vi "Arduino_Timed_Release.vi"(2 "Time to hold source ON (microseconds)":u32=1000000 format="%.0g", 3 "Time to hold source OFF (microseconds)":u32=1000000 format="%.0g", 4 "Number of cycles":u16=1) -> (0 "error out":errorcluster, 1 "Completed cycles":u16=5)   [LabVIEW 2014]
uses:
  ADAM Client/Sub VIs/ADAM Controls/Update_scan_value.ctl
  Globals/Gas_management_global.vi
  Arduino_common/Arduino_comms_Global.vi
panel:
  in  "Device index":i32
  out "bytes sent":u32=12
  out "write buffer":string
  # "(enter 0 for continuous ON)*"
  # "(enter 0 for continuous OFF)*"
  # "Paul Nathan, 18/06/2013, 02/05/2014, 12/08/2014, 03/10/2014, 10/12/2014"
  # "*until next communication. Ensure n cycles is 1 for these special operations."
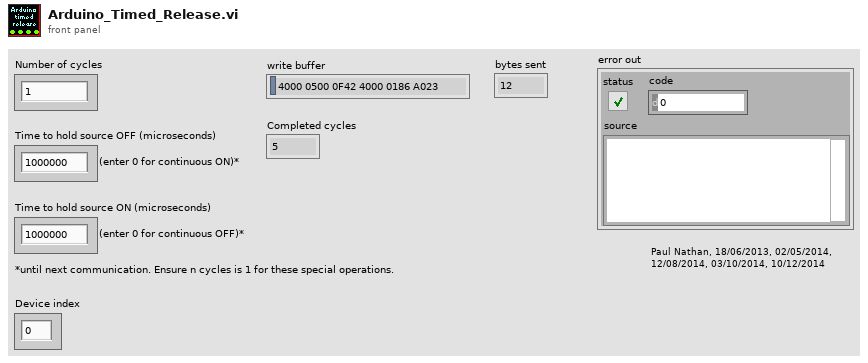
[diagram p1: front panel]
types:
  T1 = typedef "Update_scan_value.ctl" = cluster{"Channel Name":string, "New Value":dbl}
  T2 = typedef "Arduino Config & resource typedef.ctl" = cluster{"VISA resource name":refnum<visa-resource-name>, "baud rate (bps)":u32, "timeout (ms)":u32, "data bits":u16, "parity":enum16{"None", "Odd", "Even", "Mark", "Space"}, "stop bits (10: 1 bit)":u16, "flow control":u16, "termination char (hex)":u8, "Enable Termination Char":bool, "byte count":u32, "Resource locked?":bool}
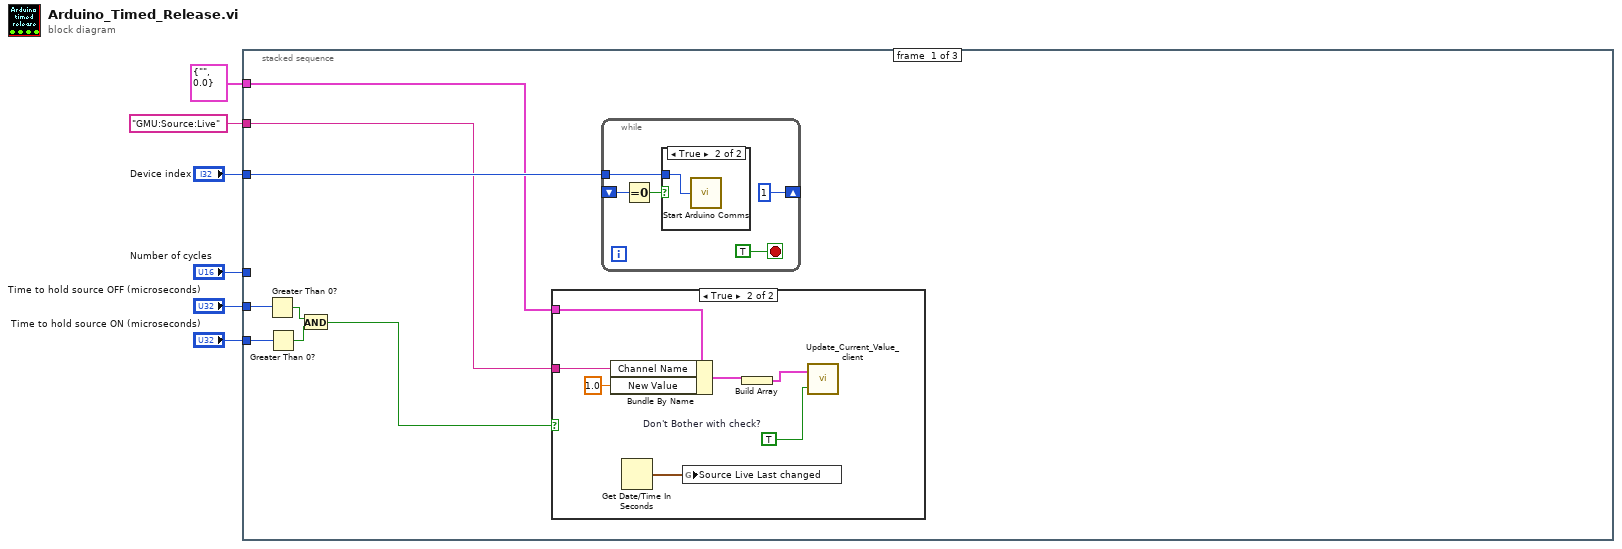
[diagram p0: block diagram]
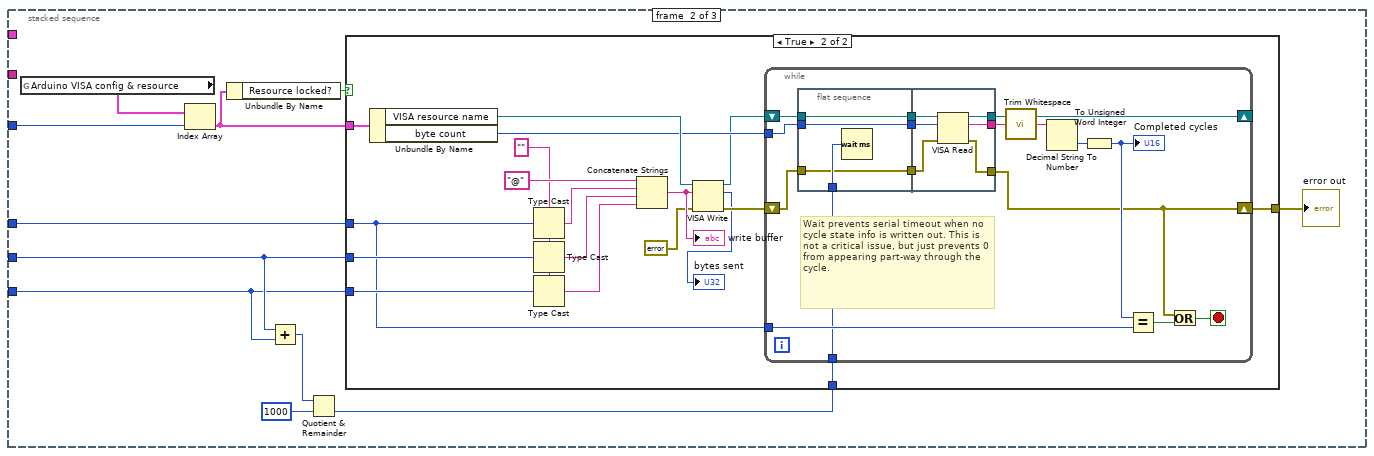
[diagram p4: hidden frame]
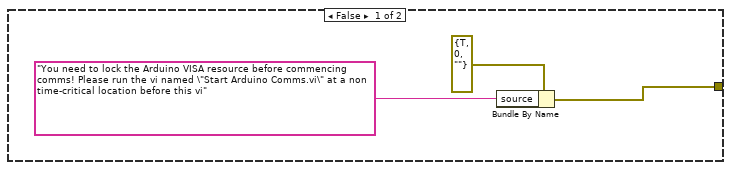
[diagram p5: hidden frame]
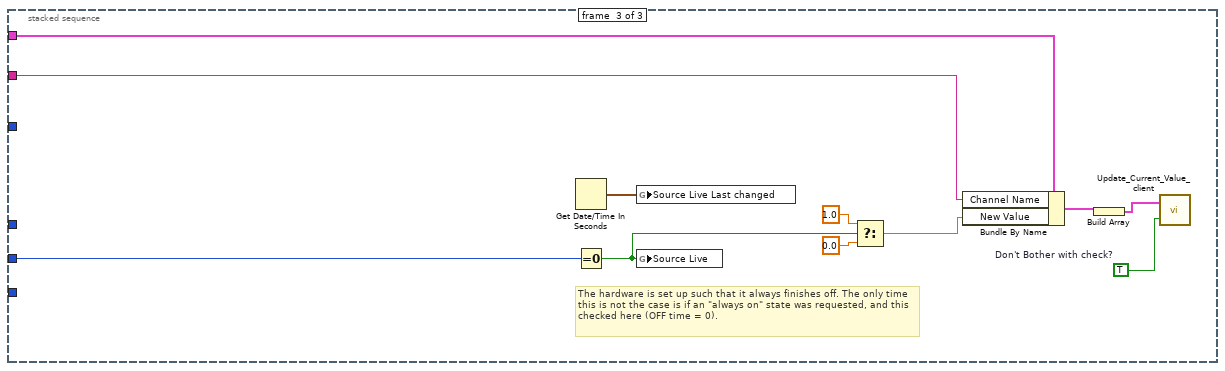
[diagram p6: hidden frame]
diagram:
  n1 = stacked-sequence {
    tunnel: "Device index" -> [w14 w31 _]
    tunnel: "Number of cycles" -> [_ w30 _]
    tunnel: "Time to hold source OFF (microseconds)" -> [w11 w29 w95]
    tunnel: "Time to hold source ON (microseconds)" -> [w10 w28 _]
    tunnel: "GMU:Source:Live" -> [w12 _ w87]
    tunnel: T1 {"Channel Name"="", "New Value"=0.0} ("Update Scan Value Cluster") -> [w13 _ w86]
    frame #0 {
      n2 = Greater Than 0?(x=w11) -> (x > 0?=w9:bool)
      n3 = Greater Than 0?(x=w10) -> (x > 0?=w8:bool)
      n4 = And(x=w9, y=w8) -> (x .and. y?=w7:bool)
      n5 = case shown="True" w7 {
        tunnel: w13 -> [_ w18]
        tunnel: w12 -> [_ w17]
        frame False {
        }
        frame True {
          w19 = TRUE  # Don't Bother with check?
          n6 = Bundle By Name(cluster=w18, "Channel Name"=w17, "New Value"=1.0) -> (w21:T1)
          n7 = Get Date/Time In Seconds() -> (seconds since 1Jan1904=w15:timestamp)
          n8 = global write "Gas_management_global.vi" "Source Live Last changed"(w15) -> ()
          n9 = Build Array(w21) -> (w20:T1[])
          n10 = call "Update_Current_Value_client.vi"("Don't Bother with check?"=w19, "Update array in"=w20) -> ()
        }
      }
      n11 = while {
        shift-right: [1] -> _
        shift-left: _ -> [w26]
        tunnel: w14 -> [w22]
        stop <- TRUE stop-if-true
        n12 = Equal To 0?(x=w26) -> (x = 0?=w25:bool)
        n13 = case shown="True" w25 {
          tunnel: w22 -> [_ w27]
          frame False {
          }
          frame True {
            n14 = call "Start Arduino Comms.vi"("Resource index"=w27) -> ()  [unwired: 1 out]
          }
        }
      }
    }
    frame #1 {
      n15 = global read "Arduino_comms_Global.vi" "Arduino VISA config & resource"() -> (w33:T2[])
      n16 = Index Array(array=w33, index=w31) -> (element=w32:T2)
      n17 = Unbundle By Name(w32) -> ("Resource locked?"=w38:bool)
      n18 = Add(x=w29, y=w28) -> (x+y=w36:u32)
      n19 = Quotient & Remainder(x=w36, y=u32 1000) -> (floor(x/y)=w34:u32)  [unwired: 1 out]
      n20 = case shown="True" w38 {
        tunnel: w32 -> [_ w57]
        tunnel: w30 -> [_ w45]
        tunnel: w29 -> [_ w55]
        tunnel: w28 -> [_ w54]
        tunnel: [w39 w47] -> w37
        tunnel: w34 -> [_ w42]
        frame False {
          n21 = Bundle By Name(cluster=errorcluster {"status"=TRUE, "code"=0, "source"=""} ("error out"), "source"="You need to lock the Arduino VISA resource before commencing comms! Please run the vi named \"Start Arduino Comms.vi\" at a non time-critical location before this vi") -> (w39:errorcluster)
        }
        frame True {
          w56 = ""
          n22 = Unbundle By Name(w57) -> ("VISA resource name"=w50:refnum<visa-resource-name>, "byte count"=w49:u32)
          n23 = Type Cast(type=w56, x=w45) -> (*(type *) &x=w53:string)
          n24 = Type Cast(type=w56, x=w55) -> (*(type *) &x=w52:string)
          n25 = Type Cast(type=w56, x=w54) -> (*(type *) &x=w51:string)
          n26 = Concatenate Strings("@", w53, w52, w51) -> (w58:string)
          "write buffer" <- w58
          n27 = VISA Write(VISA resource name=w50, write buffer=w58, error in (no error)=errorcluster {"status"=FALSE, "code"=0, "source"=""}) -> (VISA resource name out=w44:refnum<visa-resource-name>, return count=→"bytes sent":u32, error out=w48:errorcluster)
          n28 = while {
            tunnel: w49 -> [w74]
            shift-right: [w62] -> w47
            shift-left: w48 -> [w64]
            shift-right: [w73] -> _
            shift-left: w44 -> [w75]
            tunnel: w45 -> [w71]
            tunnel: w42 -> [w65]
            stop <- w60 stop-if-true
            # "Wait prevents serial timeout when no cycle state info is written out. This is not a critical issue, but just prevents 0 from appearing part-way through the cycle."
            n29 = flat-sequence {
              tunnel: w74 -> [w78]
              tunnel: w75 -> [w79]
              tunnel: [w79] -> w67
              tunnel: [w78] -> w66
              tunnel: w65 -> [w77]
              tunnel: w64 -> [w76]
              tunnel: [w76] -> w63
              tunnel: [w83] -> w73
              tunnel: [w82] -> w69
              tunnel: w67 -> [w85]
              tunnel: w66 -> [w84]
              tunnel: w63 -> [w81]
              tunnel: [w80] -> w62
              frame #0 {
                n30 = Wait (ms)(milliseconds to wait=w77) -> ()  [unwired: 1 out]
              }
              frame #1 {
                n31 = VISA Read(VISA resource name=w85, byte count=w84, error in (no error)=w81) -> (VISA resource name out=w83:refnum<visa-resource-name>, read buffer=w82:string, error out=w80:errorcluster)  [unwired: 1 out]
              }
            }
            n32 = call <vilib>:"Trim Whitespace.vi"("string"=w69) -> ("trimmed string"=w68:string)  [unwired: 1 in]
            n33 = Decimal String To Number(string=w68) -> (number=w72:i32)  [unwired: 2 in, 1 out]
            n34 = To Unsigned Word Integer(number=w72) -> (unsigned 16bit integer=w70:u16)
            "Completed cycles" <- w70
            n35 = Equal?(x=w70, y=w71) -> (x = y?=w61:bool)
            n36 = Or(x=w62, y=w61) -> (x .or. y?=w60:bool)
          }
        }
      }
      "error out" <- w37
    }
    frame #2 {
      w88 = TRUE  # Don't Bother with check?
      # "The hardware is set up such that it always finishes off. The only time this is not the case is if an \"always on\" state was requested, and this checked here (OFF time = 0)."
      n37 = Get Date/Time In Seconds() -> (seconds since 1Jan1904=w96:timestamp)
      n38 = Equal To 0?(x=w95) -> (x = 0?=w94:bool)
      n39 = global write "Gas_management_global.vi" "Source Live Last changed"(w96) -> ()
      n40 = global write "Gas_management_global.vi" "Source Live"(w94) -> ()
      n41 = Select(t=1.0, s=w94, f=0.0) -> (s? t:f=w91:dbl)
      n42 = Bundle By Name(cluster=w86, "Channel Name"=w87, "New Value"=w91) -> (w90:T1)
      n43 = Build Array(w90) -> (w89:T1[])
      n44 = call "Update_Current_Value_client.vi"("Don't Bother with check?"=w88, "Update array in"=w89) -> ()
    }
  }
